vi "Create.vi"(8 "error in":errorcluster, 10 "gRPC ID in":T1) -> (0 "error out":errorcluster, 2 "gRPC ID out":T1, 3 "measurement service out":refnum<class "IMeasurement Service.lvclass">)   [LabVIEW 2020, in "MeasurementLink Measurement Server.lvlib" / "Measurement Service V1.lvclass"]
uses:
  Measurement Service V1.lvclass
  IMeasurement Service/IMeasurement Service.lvclass
  <vilib>/gRPC/LabVIEW gRPC Library/Shared/grpcId.ctl
  C:/dev/measurementlink-labview/Source/Runtime/MeasurementLink Measurement Server/IMeasurement Service/IMeasurement Service.lvclass
  Generated/Measurement Plugin Measurement Server Internal/RPC Service/MeasurementService/MeasurementServiceBaseV1.lvclass
  Measurement Service V1.lvclass/Measurement Service V1.ctl
  <vilib>/gRPC/LabVIEW gRPC Library/grpc-lvsupport-release.lvlib
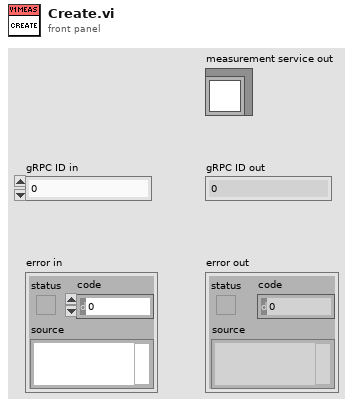
[diagram p1: front panel]
types:
  T1 = typedef "grpc-lvsupport-release.lvlib/grpcId.ctl" = u64
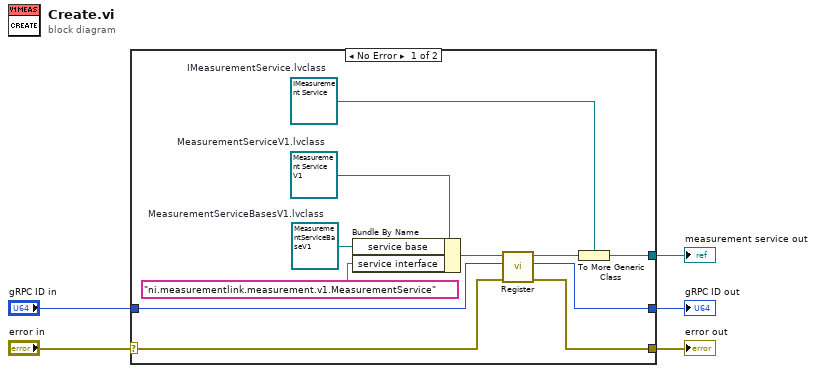
[diagram p0: block diagram]
diagram:
  n1 = case shown="No Error" "error in" {
    selector: "error in" -> [w9 w18]
    tunnel: [w8 w18] -> w4
    tunnel: [w13 _] -> w3
    tunnel: "gRPC ID in" -> [w7 w17]
    tunnel: [w6 w17] -> w1
    frame No Error {
      w12 = refnum<class "IMeasurement Service.lvclass"> refnum  # IMeasurementService.lvclass
      w15 = refnum<class "MeasurementServiceBaseV1.lvclass"> refnum  # MeasurementServiceBasesV1.lvclass
      w16 = refnum<class "Measurement Service V1.lvclass"> refnum  # MeasurementServiceV1.lvclass
      n2 = Bundle By Name(cluster=w16, "service base"=w15, "service interface"="ni.measurementlink.measurement.v1.MeasurementService") -> (w11:refnum<class "Measurement Service V1.lvclass">)
      n3 = call "Register.vi"("error in"=w9, "gRPC ID in"=w7, "measurement service v1 in"=w11) -> ("error out"=w8:errorcluster, "gRPC ID out"=w6:T1, "measurement service v1 out"=w10:refnum<class "Measurement Service V1.lvclass">)  [unwired: 6 in]
      n4 = To More Generic Class(target class=w12, reference=w10) -> (generic class reference=w13:refnum<class "IMeasurement Service.lvclass">)
    }
    frame Error {
    }
  }
  "error out" <- w4
  "measurement service out" <- w3
  "gRPC ID out" <- w1
